vi "IMAQ Reference AE.vi"(2 "error in (no error)":errorcluster, 3 "IMAQ AE States":T1) -> (0 "error out":errorcluster, 1 "Image Out":T2)   [LabVIEW 2018]
uses:
  <vilib>/vision/Image Controls.llb/IMAQ Image.ctl
  IMAQ Reference AE.ctl
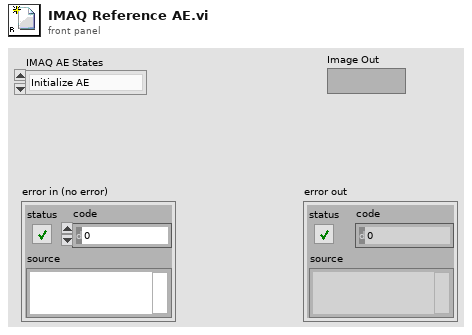
[diagram p1: front panel]
types:
  T1 = typedef "IMAQ Reference AE.ctl" = enum16{"Initialize AE", "Get IMAQ Reference", "Dispose Processing Buffer"}
  T2 = typedef "IMAQ Image.ctl" = refnum<image>
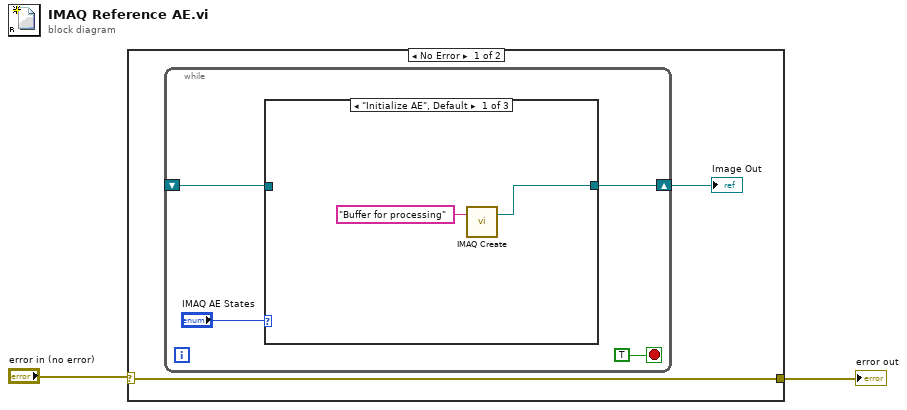
[diagram p0: block diagram]
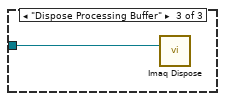
[diagram p3: hidden frame]
diagram:
  n1 = case shown="No Error" "error in (no error)" {
    selector: "error in (no error)" -> [w4 w13]
    tunnel: [w4 w13] -> w1
    frame No Error {
      n2 = while {
        shift-right: [w6] -> w3
        shift-left: _ -> [w7]
        stop <- TRUE stop-if-true
        n3 = case shown="\"Initialize AE\", Default" "IMAQ AE States" {
          tunnel: [w9 w11 _] -> w6
          tunnel: w7 -> [_ w11 w12]
          frame "Initialize AE", Default {
            n4 = call "IMAQ Create"("Image Name"="Buffer for processing") -> ("New Image"=w9:T2)  [unwired: 3 in, 2 out]
          }
          frame "Get IMAQ Reference" {
          }
          frame "Dispose Processing Buffer" {
            n5 = call "Imaq Dispose"("Image"=w12) -> ()  [unwired: 5 in, 1 out]
          }
        }
      }
      "Image Out" <- w3
    }
    frame Error {
    }
  }
  "error out" <- w1
